vi "Prevent minimum value-Bipolar.vi"(9 "No less than (+-)":sgl, 11 "Input value":sgl) -> (3 "Output value":sgl)   [LabVIEW 2017]
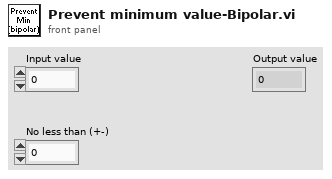
[diagram p1: front panel]
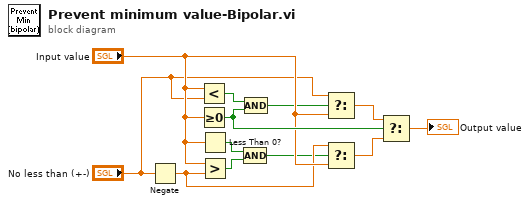
[diagram p0: block diagram]
diagram:
  n1 = Negate(x="No less than (+-)") -> (-x=w7:sgl)
  n2 = Less?(x="Input value", y="No less than (+-)") -> (x < y?=w1:bool)
  n3 = Greater Or Equal To 0?(x="Input value") -> (x >= 0?=w9:bool)
  n4 = Less Than 0?(x="Input value") -> (x < 0?=w4:bool)
  n5 = Greater?(x="Input value", y=w7) -> (0:w5:bool)
  n6 = Compound Arithmetic op=AND(w4, w5) -> (w6:bool)
  n7 = Compound Arithmetic op=AND(w1, w9) -> (w2:bool)
  n8 = Select(t="No less than (+-)", s=w2, f="Input value") -> (s? t:f=w10:sgl)
  n9 = Select(t=w7, s=w6, f="Input value") -> (s? t:f=w11:sgl)
  n10 = Select(t=w10, s=w9, f=w11) -> (s? t:f=→"Output value":sgl)
